vi "change csi for test.vi"(10 "channel estimate in":T1) -> (2 "channel estimate out":T1)   [LabVIEW 2020]
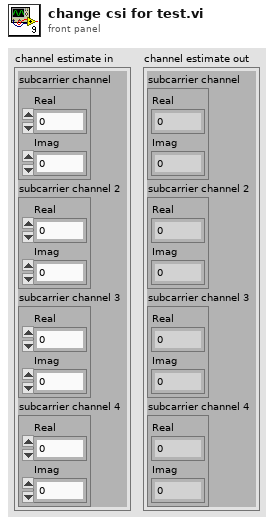
[diagram p1: front panel]
types:
  T1 = cluster{"subcarrier channel":cluster{"Real":fxp<+/-,25,4>, "Imag":fxp<+/-,25,4>}, "subcarrier channel 2":cluster{"Real":fxp<+/-,25,4>, "Imag":fxp<+/-,25,4>}, "subcarrier channel 3":cluster{"Real":fxp<+/-,25,4>, "Imag":fxp<+/-,25,4>}, "subcarrier channel 4":cluster{"Real":fxp<+/-,25,4>, "Imag":fxp<+/-,25,4>}}
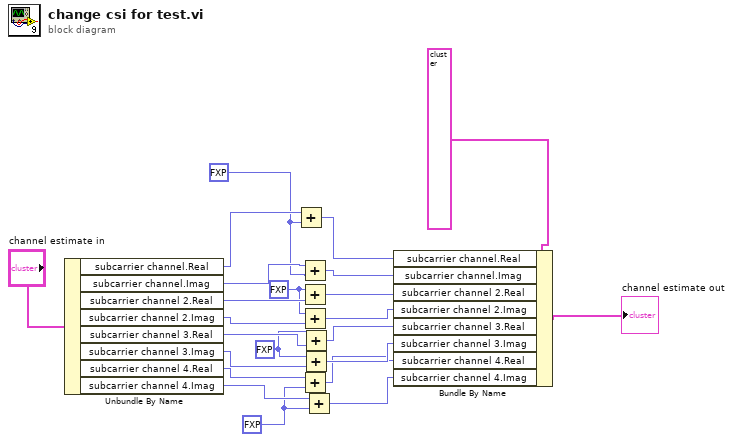
[diagram p0: block diagram]
diagram:
  w10 = fxp<+/-,25,4> 2.0 ("x")
  w11 = fxp<+/-,25,4> 1.0 ("x")
  w9 = fxp<+/-,25,4> 3.0 ("y")
  w19 = fxp<+/-,25,4> 0.0 ("y")
  n1 = Unbundle By Name("channel estimate in") -> ("subcarrier channel.Real"=w22:fxp<+/-,25,4>, "subcarrier channel.Imag"=w20:fxp<+/-,25,4>, "subcarrier channel 2.Real"=w17:fxp<+/-,25,4>, "subcarrier channel 2.Imag"=w16:fxp<+/-,25,4>, "subcarrier channel 3.Real"=w14:fxp<+/-,25,4>, "subcarrier channel 3.Imag"=w15:fxp<+/-,25,4>, "subcarrier channel 4.Real"=w13:fxp<+/-,25,4>, "subcarrier channel 4.Imag"=w12:fxp<+/-,25,4>)
  n2 = Add(x=w22, y=w19) -> (x+y=w21:fxp<+/-,25,4>)
  n3 = Add(x=w20, y=w19) -> (x+y=w18:fxp<+/-,25,4>)
  n4 = Add(x=w11, y=w17) -> (x+y=w8:fxp<+/-,25,4>)
  n5 = Add(x=w11, y=w16) -> (x+y=w7:fxp<+/-,25,4>)
  n6 = Add(x=w13, y=w9) -> (x+y=w4:fxp<+/-,25,4>)
  n7 = Add(x=w10, y=w14) -> (x+y=w6:fxp<+/-,25,4>)
  n8 = Add(x=w10, y=w15) -> (x+y=w5:fxp<+/-,25,4>)
  n9 = Add(x=w12, y=w9) -> (x+y=w3:fxp<+/-,25,4>)
  n10 = Bundle By Name(cluster=T1 {"subcarrier channel"={"Real"=0.0, "Imag"=0.0}, "subcarrier channel 2"={"Real"=0.0, "Imag"=0.0}, "subcarrier channel 3"={"Real"=0.0, "Imag"=0.0}, "subcarrier channel 4"={"Real"=0.0, "Imag"=0.0}} ("channel estimate out"), "subcarrier channel.Real"=w21, "subcarrier channel.Imag"=w18, "subcarrier channel 2.Real"=w8, "subcarrier channel 2.Imag"=w7, "subcarrier channel 3.Real"=w6, "subcarrier channel 3.Imag"=w5, "subcarrier channel 4.Real"=w4, "subcarrier channel 4.Imag"=w3) -> (→"channel estimate out":T1)
